vi "Create Group Transfers.vi"(7 "direction":T2, 8 "error in (no error)":errorcluster, 9 "Group ID":string, 10 "dsf refnum in":refnum<class "Configuration Session.lvclass">, 11 "Section Ptr":T1 format="%.0x") -> (0 "error out":errorcluster)   [LabVIEW 2017, in "Data Sharing Framework System Explorer.lvlib"]
uses:
  Data Sharing Framework System Explorer.lvlib
  Engine/DSF Core.lvlibp/Typedefs/DSF Direction.ctl
  Engine/DSF Core.lvlibp/Classes/Configuration/Configuration Session.lvclass
  <vilib>/NI Veristand/Custom Device API/Custom Device Item Ref.ctl
  Engine/DSF Core.lvlibp/Classes/Configuration/Read Group Transfer IDs.vi
  <vilib>/NI Veristand/Custom Device API/Custom Device API.lvlib
  Engine/DSF Core.lvlibp
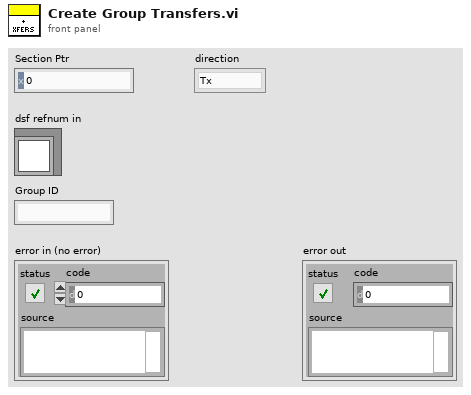
[diagram p1: front panel]
types:
  T1 = typedef "Custom Device API.lvlib/Custom Device Item Ref.ctl" = u64
  T2 = typedef "DSF Core.lvlibp/DSF Direction.ctl" = enum8{"Tx", "Rx"}
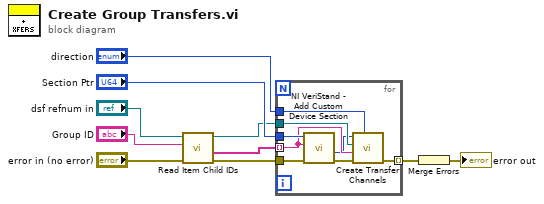
[diagram p0: block diagram]
diagram:
  n1 = call-poly "Read Item Child IDs.vi"("error in (no error)"="error in (no error)", "Group ID"="Group ID", "Configuration Session in"="dsf refnum in") -> ("error out"=w3:errorcluster, "Transfer IDs"=w2:string[], "Configuration Session out"=w1:refnum<class "Configuration Session.lvclass">)  [unwired: 5 in, 1 out]
  n2 = for {
    tunnel: w2 -> [w12] mode=indexing
    tunnel: w3 -> [w18]
    tunnel: [w16] -> w8 mode=indexing
    tunnel: "Section Ptr" -> [w17]
    tunnel: w1 -> [w14]
    tunnel: "direction" -> [w13]
    n3 = call <vilib>:"NI VeriStand - Add Custom Device Section.vi"("error in (no error)"=w18, "Section Name"=w12, "Parent Ref in"=w17) -> ("error out"=w15:errorcluster, "Section Ptr"=w11:T1)  [unwired: 5 in, 2 out]
    n4 = call "Create Transfer Channels.vi"("direction"=w13, "error in (no error)"=w15, "Transfer ID"=w12, "Refnum in"=w14, "Section Ptr"=w11) -> ("error out"=w16:errorcluster)  [unwired: 6 in]
  }
  n5 = Merge Errors(w8) -> (→"error out":errorcluster)
